vi "Initialize.vi"(8 "error in (no error)":errorcluster, 9 "Device":string, 10 "VISA Com Port":refnum<visa-resource-name>, 11 "Cypress in":refnum<class "Cypress.lvclass">) -> (0 "error out":errorcluster, 3 "Cypress out":refnum<class "Cypress.lvclass">)   [LabVIEW 2020, in "Cypress.lvclass"]
uses:
  Cypress.lvclass
  Abstract/Serial Device/Serial Device.lvclass
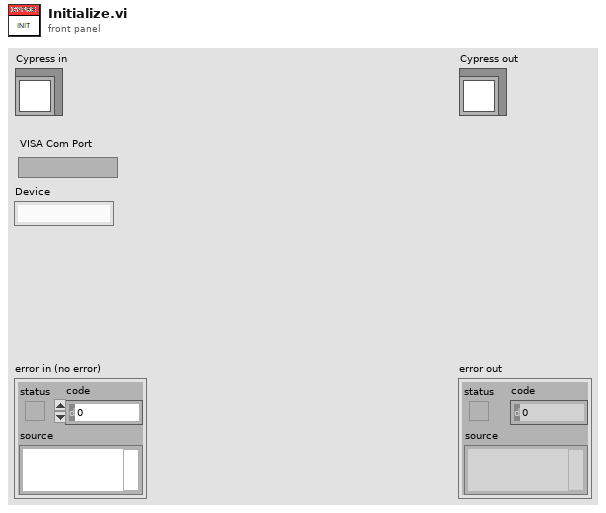
[diagram p1: front panel]
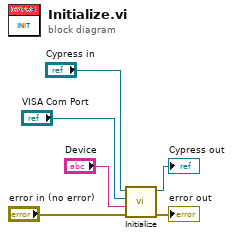
[diagram p0: block diagram]
diagram:
  n1 = call-parent "Initialize.vi"("error in (no error)"="error in (no error)", "Device"="Device", "VISA Com Port"="VISA Com Port", "Serial Device in"="Cypress in") -> ("error out"=→"error out":errorcluster, "Serial Device out"=→"Cypress out":refnum<class "Cypress.lvclass">)  [unwired: 6 in]
